vi "MU Interface Nearest Possible Frame Cycle Time.vi"(8 "error in (no error)":errorcluster, 10 "frameCycleTime_s":dbl, 11 "interfaceType":u32) -> (0 "error out (no error)":errorcluster, 3 "nearestFrameCycleTime":dbl)   [LabVIEW 2017, in "MU_3SL_interface.lvlib"]
uses:
  MU_3SL_interface.lvlib
  lib/MU_3SL_interface.dll
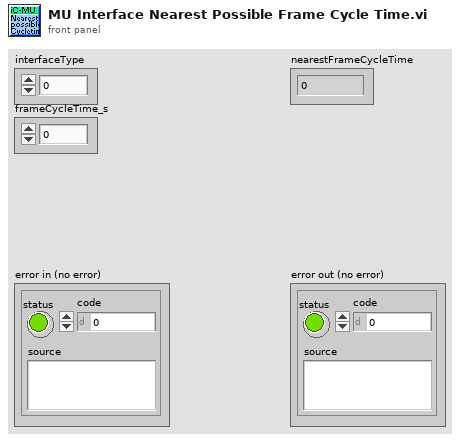
[diagram p1: front panel]
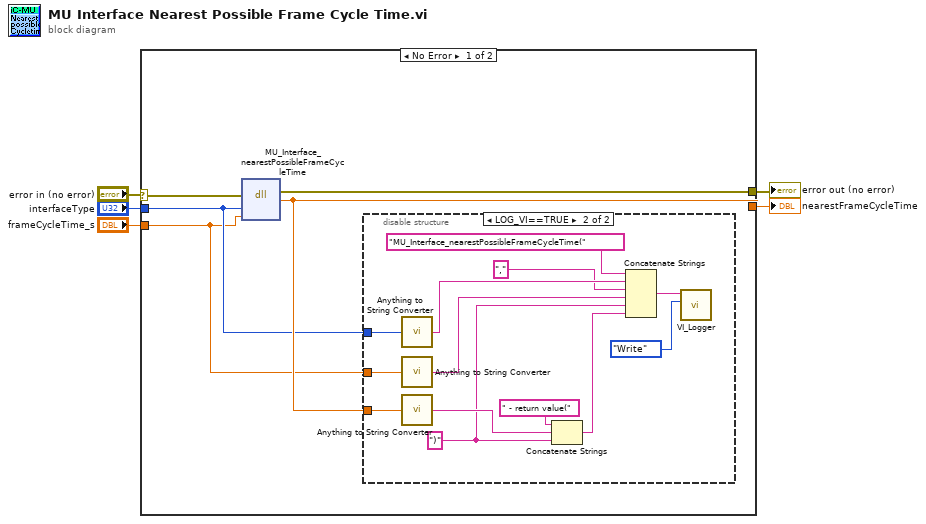
[diagram p0: block diagram]
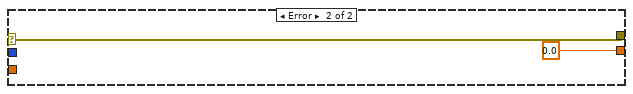
[diagram p3: hidden frame]
diagram:
  n1 = case shown="No Error" "error in (no error)" {
    selector: "error in (no error)" -> [w10 w25]
    tunnel: [w9 w25] -> w4
    tunnel: "interfaceType" -> [w7 _]
    tunnel: "frameCycleTime_s" -> [w6 _]
    tunnel: [w8 0.0 ("nearestFrameCycleTime")] -> w1
    frame No Error {
      n2 = dll-call lib="C:/Users/bes/AppData/Roaming/work/mu_9so/icsubmodules/soft_mu_3sl_master/lv_interface/lib/MU_3SL_interface**.*" fn="MU_Interface_nearestPossibleFrameCycleTime"(error in=w10, "interfaceType"=w7, "frameCycleTime_s"=w6) -> (error out=w9:errorcluster, "nearestFrameCycleTime"=w8:dbl)  [unwired: 4 in, 1 out]
      n3 = disable-structure shown="LOG_VI==TRUE" {
        disable-tunnel: w8 -> [_ w19]
        disable-tunnel: w7 -> [_ w17]
        disable-tunnel: w6 -> [_ w16]
        frame condition #0 {
        }
        frame condition #1 (active) {
          w12 = ")" ("string")
          n4 = call "Anything to String Converter.vi"("anything"=w17) -> ("String"=w15:string)
          n5 = call "Anything to String Converter.vi"("anything"=w16) -> ("String"=w14:string)
          n6 = call "Anything to String Converter.vi"("anything"=w19) -> ("String"=w18:string)
          n7 = Concatenate Strings(" - return value(" ("string"), w18, w12) -> (w11:string)
          n8 = Concatenate Strings("MU_Interface_nearestPossibleFrameCycleTime(" ("Info in"), w15, "," ("string"), w14, w12, w11) -> (w21:string)
          n9 = call "VI_Logger.vi"("Action (Read)"=enum16{"Write", "Read"}."Write", "Info in"=w21) -> ()  [unwired: 8 in, 2 out]
        }
      }
    }
    frame Error {
    }
  }
  "error out (no error)" <- w4
  "nearestFrameCycleTime" <- w1
